vi "Overlap test.vi"(8 "Stack Array":u8[][](array[numeric]), 11 "Piece Array":u8[][](array[numeric])) -> (3 "Interference":bool)   [LabVIEW 2019]
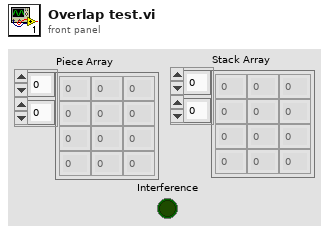
[diagram p1: front panel]
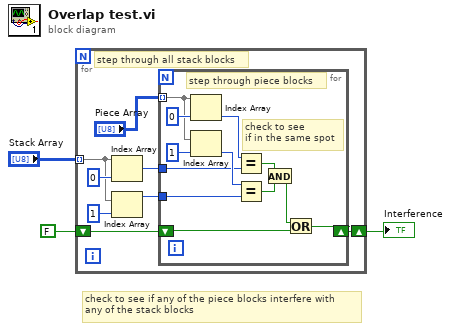
[diagram p0: block diagram]
diagram:
  # "check to see if any of the piece blocks interfere with \nany of the stack blocks"
  n1 = for {
    tunnel: "Stack Array" -> [w9] mode=indexing
    shift-right: [w4] -> w1
    shift-left: FALSE -> [w5]
    # "step through all stack blocks"
    n2 = Index Array(array=w9, index=0) -> (element=w7:u8)
    n3 = Index Array(array=w9, index=1) -> (element=w6:u8)
    n4 = for {
      tunnel: "Piece Array" -> [w21] mode=indexing
      tunnel: w7 -> [w18]
      tunnel: w6 -> [w17]
      shift-right: [w13] -> w4
      shift-left: w5 -> [w14]
      # "check to see\nif in the same spot"
      # "step through piece blocks"
      n5 = Index Array(array=w21, index=0) -> (element=w20:u8)
      n6 = Index Array(array=w21, index=1) -> (element=w19:u8)
      n7 = Equal?(x=w20, y=w18) -> (x = y?=w16:bool)
      n8 = Equal?(x=w19, y=w17) -> (x = y?=w15:bool)
      n9 = And(x=w16, y=w15) -> (x .and. y?=w12:bool)
      n10 = Or(x=w12, y=w14) -> (x .or. y?=w13:bool)
    }
  }
  "Interference" <- w1
